vi "Main.vi"() -> ()   [LabVIEW 2017, in "VisitorPatternDemo.lvclass"]
uses:
  VisitorPatternDemo.lvclass
  Dot Class/Dot.lvclass
  C:/Users/fflores/Documents/LabVIEW-Open-Projects/LabIVEW OOP Design Patterns/Visitor Pattern/Shape Class/Shape.lvclass
  Circle Class/Circle.lvclass
  Rectangle Class/Rectangle.lvclass
  CompoundShape Class/CompoundShape.lvclass
  XMLExportVisitor Class/XMLExportVisitor.lvclass
panel:
  out "XML String Exported":string
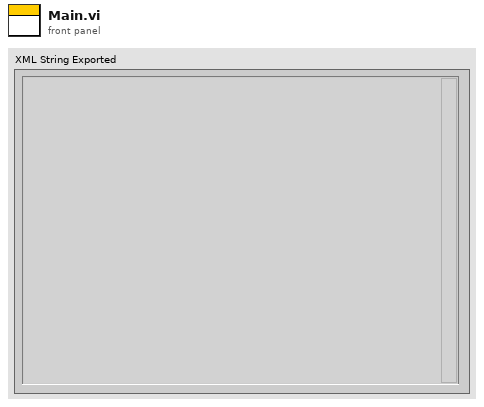
[diagram p1: front panel]
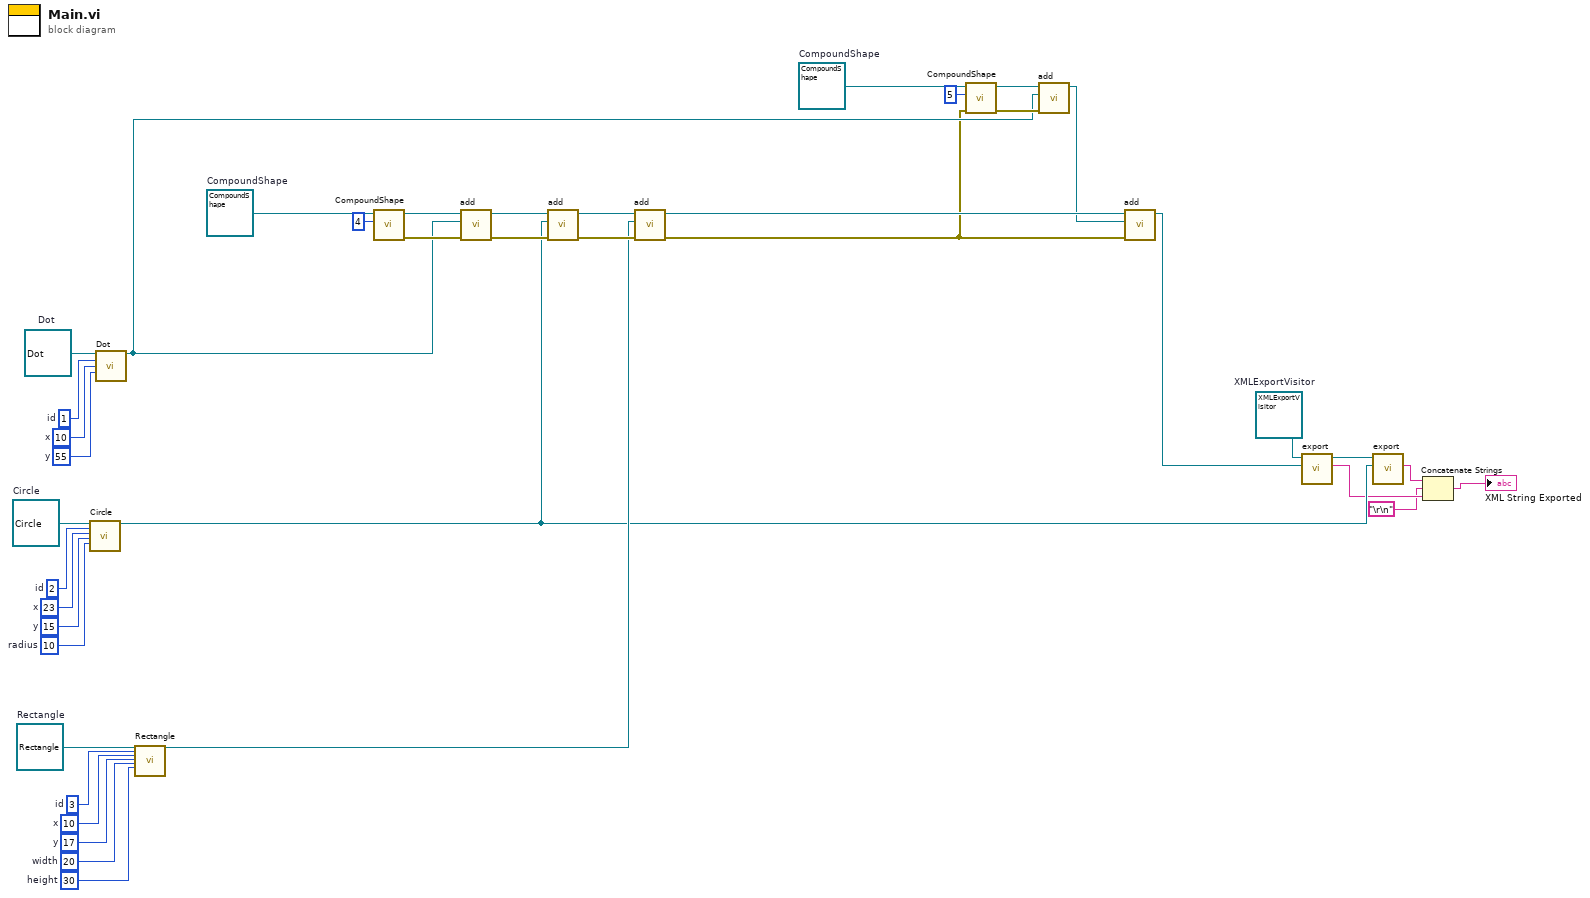
[diagram p0: block diagram]
diagram:
  w11 = refnum<class "XMLExportVisitor.lvclass"> refnum  # XMLExportVisitor
  w15 = refnum<class "CompoundShape.lvclass"> refnum  # CompoundShape
  w26 = 30  # height
  w27 = 20  # width
  w28 = 17  # y
  w29 = 10  # x
  w30 = 3  # id
  w32 = 10  # radius
  w33 = 15  # y
  w34 = 23  # x
  w35 = 2  # id
  w25 = refnum<class "CompoundShape.lvclass"> refnum  # CompoundShape
  w31 = refnum<class "Rectangle.lvclass"> refnum  # Rectangle
  w36 = refnum<class "Circle.lvclass"> refnum  # Circle
  w37 = 55  # y
  w38 = 10  # x
  w39 = 1  # id
  w40 = refnum<class "Dot.lvclass"> refnum  # Dot
  n1 = call "Circle.vi"("Circle in"=w36, "id"=w35, "x"=w34, "y"=w33, "radius"=w32) -> ("Circle out"=w8:refnum<class "Circle.lvclass">)  [unwired: 13 in, 1 out]
  n2 = call "Dot.vi"("Dot in"=w40, "id"=w39, "x"=w38, "y"=w37) -> ("Dot out"=w12:refnum<class "Dot.lvclass">)  [unwired: 10 in, 1 out]
  n3 = call "Rectangle.vi"("Rectangle in"=w31, "id"=w30, "x"=w29, "y"=w28, "width"=w27, "height"=w26) -> ("Rectangle out"=w17:refnum<class "Rectangle.lvclass">)  [unwired: 20 in, 1 out]
  n4 = call "CompoundShape.vi"("id"=4, "CompoundShape in"=w25) -> ("error out"=w22:errorcluster, "CompoundShape out"=w23:refnum<class "CompoundShape.lvclass">)  [unwired: 8 in]
  n5 = call "add.vi"("error in (no error)"=w22, "Shape"=w12, "CompoundShape in"=w23) -> ("error out"=w20:errorcluster, "CompoundShape out"=w21:refnum<class "CompoundShape.lvclass">)  [unwired: 7 in]
  n6 = call "add.vi"("error in (no error)"=w20, "Shape"=w8, "CompoundShape in"=w21) -> ("error out"=w18:errorcluster, "CompoundShape out"=w19:refnum<class "CompoundShape.lvclass">)  [unwired: 7 in]
  n7 = call "add.vi"("error in (no error)"=w18, "Shape"=w17, "CompoundShape in"=w19) -> ("error out"=w3:errorcluster, "CompoundShape out"=w4:refnum<class "CompoundShape.lvclass">)  [unwired: 7 in]
  n8 = call "CompoundShape.vi"("error in (no error)"=w3, "id"=5, "CompoundShape in"=w15) -> ("error out"=w13:errorcluster, "CompoundShape out"=w14:refnum<class "CompoundShape.lvclass">)  [unwired: 7 in]
  n9 = call "add.vi"("error in (no error)"=w13, "Shape"=w12, "CompoundShape in"=w14) -> ("CompoundShape out"=w2:refnum<class "CompoundShape.lvclass">)  [unwired: 7 in, 1 out]
  n10 = call "add.vi"("error in (no error)"=w3, "Shape"=w2, "CompoundShape in"=w4) -> ("CompoundShape out"=w1:refnum<class "CompoundShape.lvclass">)  [unwired: 7 in, 1 out]
  n11 = call "export.vi"("Shape"=w1, "XMLExportVisitor in"=w11) -> ("String"=w6:string, "XMLExportVisitor out"=w10:refnum<class "XMLExportVisitor.lvclass">)  [unwired: 7 in, 1 out]
  n12 = call "export.vi"("Shape"=w8, "XMLExportVisitor in"=w10) -> ("String"=w9:string)  [unwired: 7 in, 2 out]
  n13 = Concatenate Strings(w9, "\r\n", w6) -> (→"XML String Exported":string)
